vi "补码给定1.vi"(11 "数值":i16) -> (2 "字符串 2":string, 3 "十六进制整型字符串":string)   [LabVIEW 2012]
panel:
  out "连接的字符串 3":string
  out "x+y 2":i16 format="%x"
  out "布尔数组":bool[](array[boolean])
  out "数值 2":i16 format="%b"
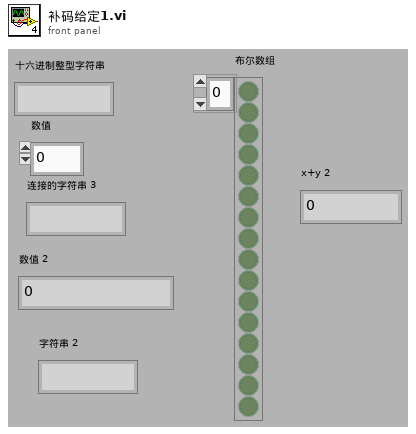
[diagram p1: front panel]
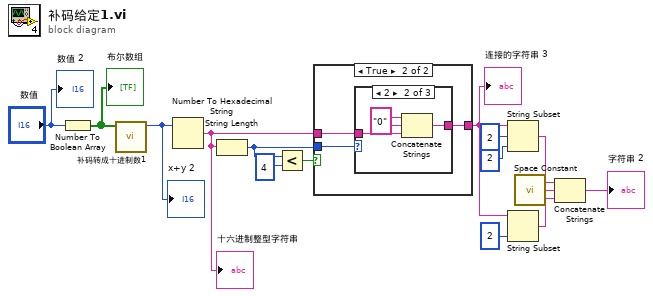
[diagram p0: block diagram]
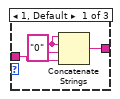
[diagram p3: hidden frame]
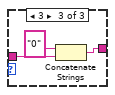
[diagram p4: hidden frame]
diagram:
  n1 = Number To Boolean Array(number="数值") -> (Boolean array=w2:bool[])
  "布尔数组" <- w2
  n2 = call "补码转成十进制数1.vi"("数组"=w2) -> ("x+y 2"=w1:i16)  [unwired: 10 in]
  "x+y 2" <- w1
  n3 = Number To Hexadecimal String(2:w1) -> (0:w3:string)  [unwired: 1 out]
  "十六进制整型字符串" <- w3
  n4 = String Length(string=w3) -> (length=w5:i32)
  n5 = Less?(x=w5, y=4) -> (x < y?=w6:bool)
  n6 = case shown="True" w6 {
    tunnel: w3 -> [w16 w19]
    tunnel: w5 -> [_ w18]
    tunnel: [w16 w17] -> w4
    frame False {
    }
    frame True {
      n7 = case shown="2" w18 {
        tunnel: w19 -> [w22 w25 w28]
        tunnel: [w20 w23 w26] -> w17
        frame 1, Default {
          w21 = "0" ("字符串")
          n8 = Concatenate Strings(w21, w21, w21, w22) -> (w20:string)
        }
        frame 2 {
          w24 = "0" ("字符串")
          n9 = Concatenate Strings(w24, w24, w25) -> (w23:string)
        }
        frame 3 {
          n10 = Concatenate Strings("0" ("字符串"), w28) -> (w26:string)
        }
      }
    }
  }
  "连接的字符串 3" <- w4
  n11 = String Subset(string=w4, offset (0)=2 ("偏移量(0)"), length (rest)=2 ("长度（剩余）")) -> (substring=w10:string)
  n12 = String Subset(string=w4, length (rest)=2 ("长度（剩余）")) -> (substring=w8:string)  [unwired: 1 out]
  n13 = call <vilib>:"Space Constant.vi"() -> ("String"=w9:string)
  n14 = Concatenate Strings(w10, w9, w8) -> (→"字符串 2":string)
  "数值 2" <- "数值"
